vi "Msg Get Message.vi"(0 "queue":refnum<queue>, 1 "timeout in ms (-1)":i32=-1, 3 "error in (no error)":errorcluster) -> (4 "Response Notifier":refnum<notifier>, 5 "queue out":refnum<queue>, 6 "Message":string, 7 "Data":variant, 8 "error out":errorcluster)   [LabVIEW 2014]
doc: "Retrieve the next message in the message queue (created by Msg Create Message Queue) or block until a message is received or the timeout has expired. If the timeout expires, the Message output will yield a string \"timeout\" and Data will be empty.\n\nThis is part of the Msg suite, intended to make messaging architectures in LabVIEW\nSee the template \"Message Based Application Template.vi\" for normal usage.\n\nCopyright 2005-2016 Jason Sommerville\n\nThis VI may be freely used, modified or distributed under the BSD license."
uses:
  Message Cluster.ctl
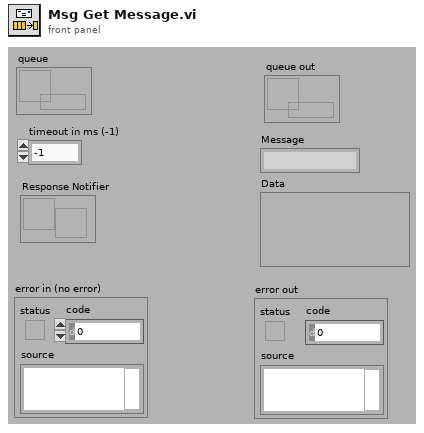
[diagram p1: front panel]
types:
  T1 = typedef "Message Cluster.ctl" = cluster{"Message":string, "Data":variant, "Response Notifier":refnum<notifier>}
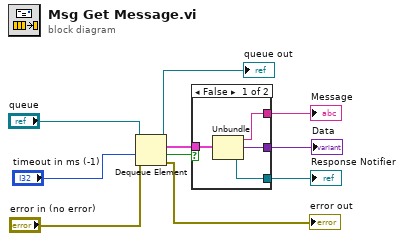
[diagram p0: block diagram]
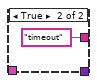
[diagram p2: hidden frame]
diagram:
  n1 = Dequeue Element(queue="queue", timeout in ms (-1)="timeout in ms (-1)", error in (no error)="error in (no error)") -> (queue out=→"queue out":refnum<queue>, element=w5:T1, timed out?=w1:bool, error out=→"error out":errorcluster)
  n2 = case shown="False" w1 {
    tunnel: [w14 _] -> w9
    tunnel: [w13 "timeout" ("Message")] -> w8
    tunnel: w5 -> [w12 _]
    tunnel: [w11 _] -> w2
    frame False {
      n3 = Unbundle(w12) -> ("Message"=w13:string, "Data"=w14:variant, "Response Notifier"=w11:refnum<notifier>)
    }
    frame True {
    }
  }
  "Data" <- w9
  "Message" <- w8
  "Response Notifier" <- w2
